vi "test_sup.vi"() -> ()   [LabVIEW 2015]
panel:
  out "FPGA Reference":refnum<k20>
  out "Time (ns)":dbl
  out "Offset":dbl(knob) scale=0.0..10.0
  out "PPS":bool
  out "Timekeeper Locked":bool
  out "FPGA Interface":refnum<k20>
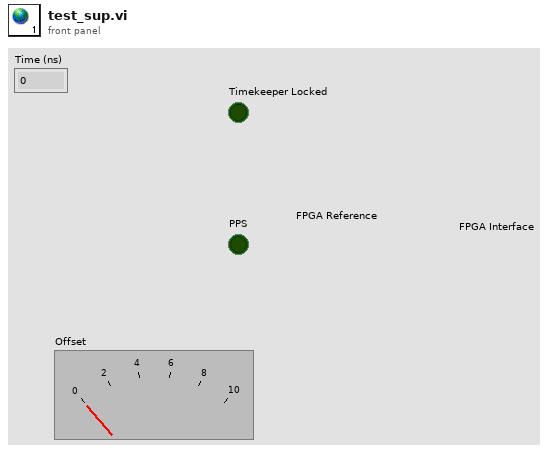
[diagram p1: front panel]
diagram:
